vi "Update Fire.vi"(8 "error in (no error)":errorcluster, 10 "Fire":dbl format="%.2f C°", 11 "Cooker Actor Logic in":refnum<class "Cooker Actor Logic.lvclass">) -> (0 "error out":errorcluster, 3 "Cooker Actor Logic out":refnum<class "Cooker Actor Logic.lvclass">)   [LabVIEW 2024, in "Cooker Actor Logic.lvlib" / "Cooker Actor Logic.lvclass"]
uses:
  Cooker Actor Logic.lvclass
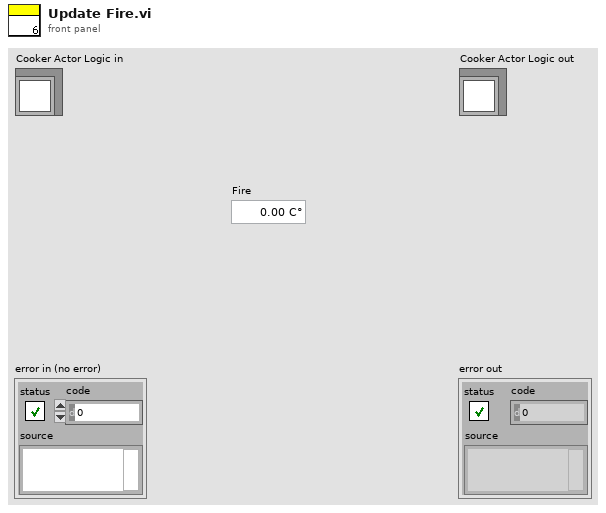
[diagram p1: front panel]
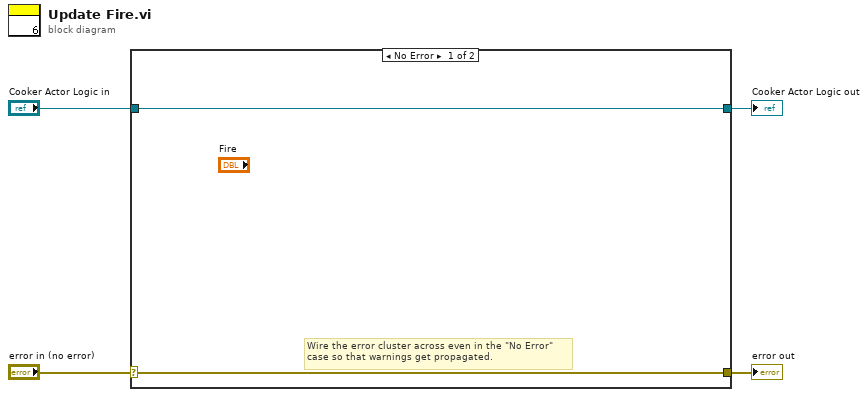
[diagram p0: block diagram]
diagram:
  n1 = case shown="No Error" "error in (no error)" {
    selector: "error in (no error)" -> [w5 w8]
    tunnel: [w5 w8] -> w3
    tunnel: [w6 w7] -> w1
    tunnel: "Cooker Actor Logic in" -> [w6 w7]
    frame No Error {
      # "Wire the error cluster across even in the \"No Error\"\ncase so that warnings get propagated."
    }
    frame Error {
    }
  }
  "error out" <- w3
  "Cooker Actor Logic out" <- w1
